vi "Query System Mode.vi"(8 "error in (no error)":errorcluster, 11 "VISA resource name":refnum<visa-resource-name>) -> (0 "error out":errorcluster, 2 "System Mode":i32(ring) items=["Local", "Remote", "Remote with Lock", "Voltage", "Current", "Dual"], 3 "VISA resource name out":refnum<visa-resource-name>)   [LabVIEW 2018, in "XP Power PLS600.lvlib"]
doc: "Queries the presently selected Control Source. Control Sources include: Local control from the front panel of the instrument, Remote control over the SCPI interface with limited front panel functionality, Remote with Lock control over the SCPI interface with no front panel capability, Analog Voltage Control where the voltage setpoint is determined by the analog voltage input, Analog Current Control where the current setpoint is determined by the analog current input, or Dual Analog Control where the voltage and current setpoint are determined by their respective analog inputs."
uses:
  XP Power PLS600.lvlib
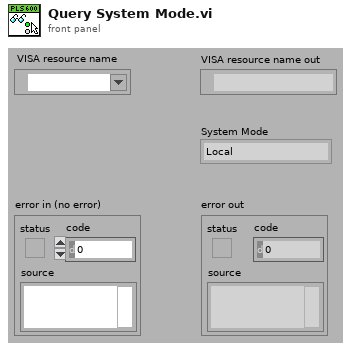
[diagram p1: front panel]
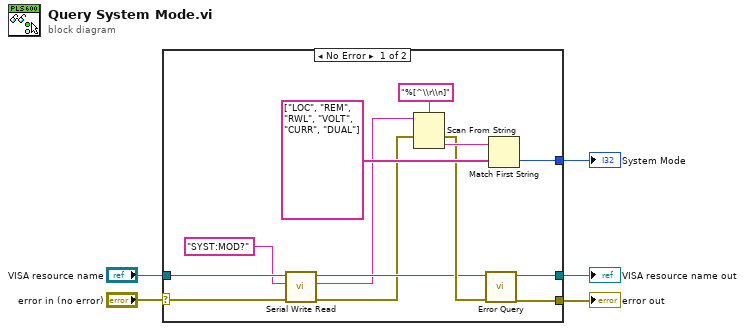
[diagram p0: block diagram]
diagram:
  n1 = case shown="No Error" "error in (no error)" {
    selector: "error in (no error)" -> [w6 w20]
    tunnel: [w18 w19] -> w5
    tunnel: [w17 w20] -> w4
    tunnel: [w15 _] -> w3
    tunnel: "VISA resource name" -> [w11 w19]
    frame No Error {
      n2 = call "Serial Write Read.vi"("error in (no error)"=w6, "Write Buffer"="SYST:MOD?", "VISA resource name"=w11) -> ("error out"=w7:errorcluster, "Read Buffer"=w8:string, "VISA resource name out"=w9:refnum<visa-resource-name>)  [unwired: 6 in]
      n3 = Scan From String(format string="%[^\\r\\n]", input string=w8, error in=w7) -> (error out=w12:errorcluster, output 1=w13:string)  [unwired: 2 in, 2 out]
      n4 = call "Error Query.vi"("error in (no error)"=w12, "VISA resource name"=w9) -> ("error out"=w17:errorcluster, "VISA resource name out"=w18:refnum<visa-resource-name>)  [unwired: 6 in, 2 out]
      n5 = Match First String(2:string[] ["LOC", "REM", "RWL", "VOLT", "CURR", "DUAL"], 3:w13) -> (0:w15:i32)  [unwired: 1 out]
    }
    frame Error {
    }
  }
  "System Mode" <- w3
  "VISA resource name out" <- w5
  "error out" <- w4
